vi "Initialize.vi"(10 "Symbol Folder Path":path, 11 "Tree in":refnum<class "Tree.lvclass">) -> (3 "Tree out":refnum<class "Tree.lvclass">)   [LabVIEW 2022 SP3, in "Tree.lvclass"]
uses:
  Tree.lvclass
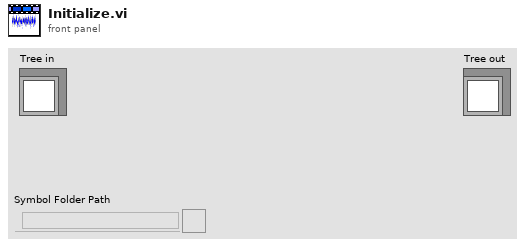
[diagram p1: front panel]
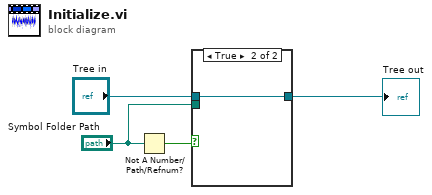
[diagram p0: block diagram]
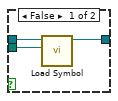
[diagram p2: hidden frame]
diagram:
  n1 = Not A Number/Path/Refnum?(number/path/refnum="Symbol Folder Path") -> (NaN/Path/Refnum?=w2:bool)
  n2 = case shown="True" w2 {
    tunnel: "Tree in" -> [w7 w8]
    tunnel: [w6 w8] -> w3
    tunnel: "Symbol Folder Path" -> [w5 _]
    frame False {
      n3 = call-dynamic "Load Symbol.vi"("Symbol Folder Path"=w5, "Tree in"=w7) -> ("Tree out"=w6:refnum<class "Tree.lvclass">)  [unwired: 9 in]
    }
    frame True {
    }
  }
  "Tree out" <- w3
